vi "Top.vi"(8 "error in (no error)":errorcluster, 9 "reposition window":bool, 10 "window position":cluster{"Left":i16, "Top":i16}, 11 "Thread in":refnum<class "Thread.lvclass">) -> (0 "error":errorcluster, 3 "Thread out":refnum<class "Thread.lvclass">)   [LabVIEW 2017, in "DSF Core.lvlib" / "Thread.lvclass"]
uses:
  Thread.lvclass
  Thread State.ctl
  Thread.lvclass/Thread.ctl
  <vilib>/Platform/TimedLoop/XDataNode/timing_clust.ctl
  <vilib>/Platform/TimedLoop/XDataNode/nitl_modes.ctl
  <vilib>/Platform/TimedLoop/XDataNode/wakeup.ctl
  <vilib>/platform/TimedLoop/XDataNode/XDataNode.xnode
  <vilib>/Platform/TimedLoop/XDataNode/XDNodeRunTimeDep.lvlib
panel:
  out "Priority":u16
  out "Processor":i32
  out "Run Count":i32
  out "State":T1
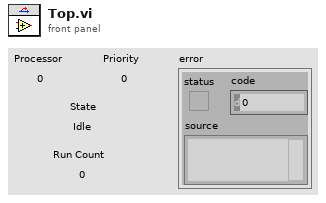
[diagram p1: front panel]
types:
  T1 = typedef "DSF Core.lvlib/Thread.lvclass/Thread State.ctl" = enum8{"Idle", "Running", "Error", "Shut Down"}
  T2 = typedef "XDNodeRunTimeDep.lvlib/timing_clust.ctl" = cluster{"Expected End [f-1]":u64, "Actual End [f-1]":u64, "Finished Late? [f-1]":bool, "Expected End [i-1]":u64, "Actual End [i-1]":u64, "Finished Late? [i-1]":bool, "Expected Start [i]":u64, "Actual Start [i]":u64, "Expected Start [f]":u64, "Actual Start [f]":u64, "Source Name":string, "Structure Name":string, "Period":i64, "Deadline":i64, "Offset":i64, "Start":i64, "Priority":i32, "Timeout":i32, "Mode":T3, "Wakeup Reason":T4, "Error":errorcluster, "Source Type":string, "Secondary Source Type":string, "Global End Time":u64, "Global Start Time":u64, "Frame Duration":u64, "Iteration Duration":u64, "Assigned CPU":i32, "I/O Scan Engine Mode":u32}
  T3 = typedef "XDNodeRunTimeDep.lvlib/nitl_modes.ctl" = enum32{"No Change", "Process missed periods, maintain original phase", "Discard missed periods, maintain original phase", "Process missed periods, ignore original phase", "Discard missed periods, ignore original phase"}
  T4 = typedef "XDNodeRunTimeDep.lvlib/wakeup.ctl" = enum32{"Normal", "Aborted", "Asynchronous wakeup", "Timing source error", "Timed loop error", "Timeout"}
  T5 = typedef "DSF Core.lvlib/Thread.lvclass/Thread Command.ctl" = enum8{"Run", "Shutdown"}
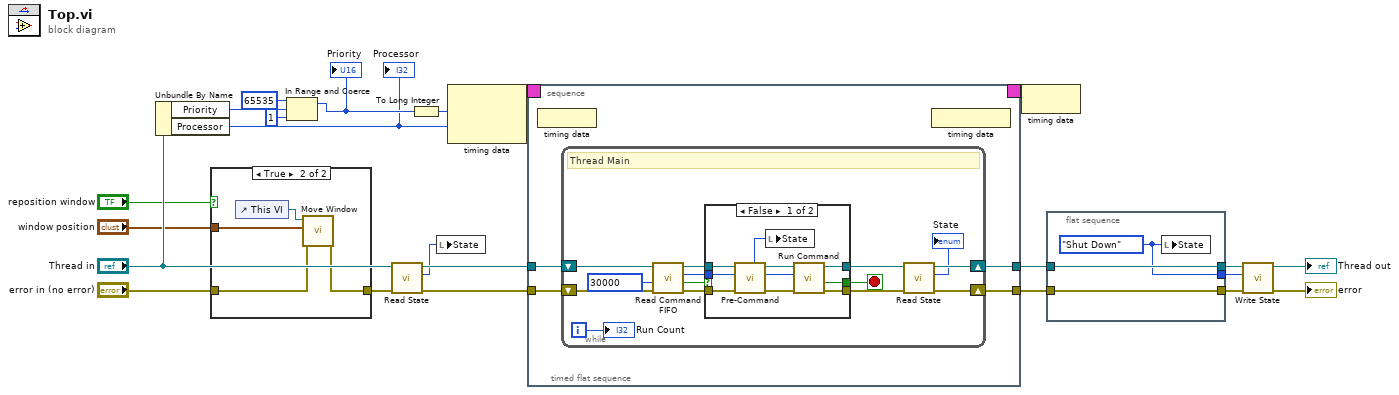
[diagram p0: block diagram]
diagram:
  n1 = Unbundle By Name("Thread in") -> ("Priority"=w8:u16, "Processor"=w6:i32)
  "Processor" <- w6
  n2 = case shown="True" "reposition window" {
    tunnel: "error in (no error)" -> [w24 w28]
    tunnel: [w24 w27] -> w4
    tunnel: "window position" -> [_ w26]
    frame False {
    }
    frame True {
      n3 = control-ref of="This VI"() -> (w25:refnum<vi>)
      n4 = call "Move Window.vi"("error in (no error)"=w28, "window position"=w26, "VI Ref"=w25) -> ("error out"=w27:errorcluster)  [unwired: 8 in]
    }
  }
  n5 = In Range and Coerce(upper limit=u16 65535, x=w8, lower limit=u16 1) -> (coerced(x)=w7:u16)  [unwired: 1 out]
  "Priority" <- w7
  n6 = call "Read State.vi"("error in (no error)"=w4, "Thread in"="Thread in") -> ("error out"=w13:errorcluster, "state"=w12:T1, "Thread out"=w14:refnum<class "Thread.lvclass">)  [unwired: 7 in]
  n7 = To Long Integer(number=w7) -> (32bit integer=w11:i32)
  n8 = local write "State"(w12) -> ()
  n9 = node-c288(w11, w6) -> (w23:T2)
  n10 = timed-sequence {
    timing: w23 -> [_]
    timing-out: [_] -> w22
    tunnel: w13 -> [w32]
    tunnel: [w31] -> w17
    tunnel: [w30] -> w18
    tunnel: w14 -> [w29]
    n11 = timed-flat-sequence {
      tunnel: w32 -> [w33]
      tunnel: [w36] -> w31
      tunnel: [w35] -> w30
      tunnel: w29 -> [w34]
      n12 = node-c288() -> ()  [unwired: 1 in]
      n13 = while {
        shift-right: [w40] -> w35
        shift-left: w34 -> [w50]
        shift-right: [w39] -> w36
        shift-left: w33 -> [w43]
        i -> [w37]
        stop <- w44 stop-if-true
        # "Thread Main"
        n14 = call "Read Command FIFO.vi"("error in (no error)"=w43, "timeout in ms (0)"=30000, "Thread in"=w50) -> ("error out"=w48:errorcluster, "timed out?"=w45:bool, "command"=w47:T5, "Thread out"=w49:refnum<class "Thread.lvclass">)  [unwired: 4 in, 1 out]
        n15 = case shown="False" w45 {
          selector: w45 -> [_ w61]
          tunnel: [w60 w62] -> w41
          tunnel: [w59 w63] -> w42
          tunnel: w49 -> [w56 w63]
          tunnel: w48 -> [w57 w62]
          tunnel: w47 -> [w55 _]
          tunnel: [w58 w61] -> w44
          frame False {
            n16 = call "Pre-Command.vi"("error in (no error)"=w57, "command in"=w55, "Thread in"=w56) -> ("error out"=w52:errorcluster, "command out"=w54:T5, "Thread out"=w53:refnum<class "Thread.lvclass">, "state"=w51:T1)  [unwired: 5 in]
            n17 = local write "State"(w51) -> ()
            n18 = call "Run Command.vi"("error in (no error)"=w52, "command"=w54, "Thread in"=w53) -> ("error out"=w60:errorcluster, "shutdown?"=w58:bool, "Thread out"=w59:refnum<class "Thread.lvclass">)  [unwired: 6 in]
          }
          frame True {
          }
        }
        n19 = call "Read State.vi"("error in (no error)"=w41, "Thread in"=w42) -> ("error out"=w39:errorcluster, "state"=→"State":T1, "Thread out"=w40:refnum<class "Thread.lvclass">)  [unwired: 7 in]
        "Run Count" <- w37
      }
      n20 = node-c288() -> ()  [unwired: 1 out]
    }
  }
  n21 = node-c288(w22) -> ()
  n22 = flat-sequence {
    tunnel: [w66] -> w19
    tunnel: w18 -> [w67]
    tunnel: w17 -> [w68]
    tunnel: [w68] -> w16
    tunnel: [w67] -> w15
    frame #0 {
      w66 = Thread_State."Shut Down" ("state")
      n23 = local write "State"(w66) -> ()
    }
  }
  n24 = call "Write State.vi"("error in (no error)"=w16, "state"=w19, "Thread in"=w15) -> ("error out"=→"error":errorcluster, "Thread out"=→"Thread out":refnum<class "Thread.lvclass">)  [unwired: 7 in]
